vi "ExecuteCommand.vi"(10 "Params":string[][](array[string]), 11 "Command":string) -> ()   [LabVIEW 2019]
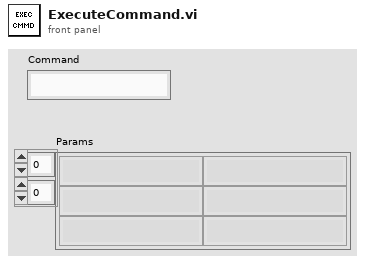
[diagram p1: front panel]
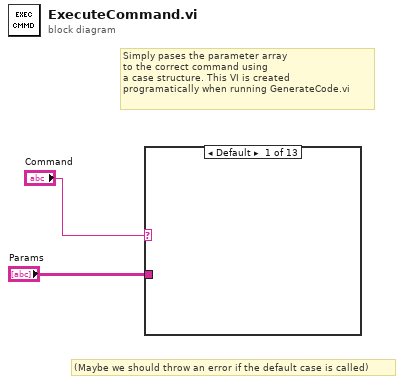
[diagram p0: block diagram]
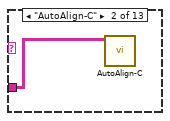
[diagram p2: hidden frame]
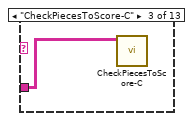
[diagram p3: hidden frame]
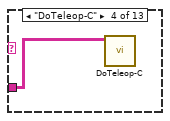
[diagram p4: hidden frame]
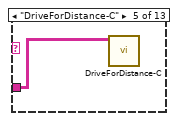
[diagram p5: hidden frame]
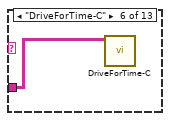
[diagram p6: hidden frame]
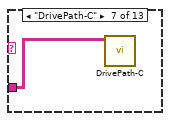
[diagram p7: hidden frame]
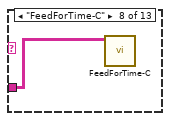
[diagram p8: hidden frame]
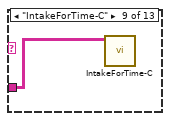
[diagram p9: hidden frame]
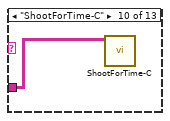
[diagram p10: hidden frame]
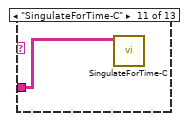
[diagram p11: hidden frame]
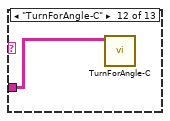
[diagram p12: hidden frame]
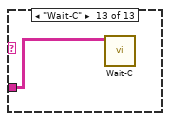
[diagram p13: hidden frame]
diagram:
  # "(Maybe we should throw an error if the default case is called)"
  # "Simply pases the parameter array\nto the correct command using\na case structure. This VI is created\nprogramatically when running GenerateCode.vi"
  n1 = case shown="Default" "Command" {
    tunnel: "Params" -> [_ w3 w4 w5 w6 w7 w8 w9 w10 w11 w12 w13 w14]
    frame Default {
    }
    frame "AutoAlign-C" {
      n2 = call "AutoAlign-C.vi"("Params"=w3) -> ()  [unwired: 11 in]
    }
    frame "CheckPiecesToScore-C" {
      n3 = call "CheckPiecesToScore-C.vi"("Params"=w4) -> ()  [unwired: 11 in]
    }
    frame "DoTeleop-C" {
      n4 = call "DoTeleop-C.vi"("Params"=w5) -> ()  [unwired: 11 in]
    }
    frame "DriveForDistance-C" {
      n5 = call "DriveForDistance-C.vi"("Params"=w6) -> ()  [unwired: 11 in]
    }
    frame "DriveForTime-C" {
      n6 = call "DriveForTime-C.vi"("Params"=w7) -> ()  [unwired: 11 in]
    }
    frame "DrivePath-C" {
      n7 = call "DrivePath-C.vi"("Params"=w8) -> ()  [unwired: 11 in]
    }
    frame "FeedForTime-C" {
      n8 = call "FeedForTime-C.vi"("Params"=w9) -> ()  [unwired: 11 in]
    }
    frame "IntakeForTime-C" {
      n9 = call "IntakeForTime-C.vi"("Params"=w10) -> ()  [unwired: 11 in]
    }
    frame "ShootForTime-C" {
      n10 = call "ShootForTime-C.vi"("Params"=w11) -> ()  [unwired: 11 in]
    }
    frame "SingulateForTime-C" {
      n11 = call "SingulateForTime-C.vi"("Params"=w12) -> ()  [unwired: 11 in]
    }
    frame "TurnForAngle-C" {
      n12 = call "TurnForAngle-C.vi"("Params"=w13) -> ()  [unwired: 11 in]
    }
    frame "Wait-C" {
      n13 = call "Wait-C.vi"("Params"=w14) -> ()  [unwired: 11 in]
    }
  }
